vi "DequeueMessage.vi"(7 "Timeout (-1 ms)":i32=-1, 8 "error in":errorcluster, 11 "PriorityMessageQueue":refnum<class "PriorityMessageQueue.lvclass">) -> (0 "error out":errorcluster, 1 "Message out":refnum<class "Message.lvclass">, 2 "Message Name":string, 3 "PriorityMessageQueue out":refnum<class "PriorityMessageQueue.lvclass">, 4 "Timed Out?":bool)   [LabVIEW 2009, in "LapDog.Messaging.v2.lvlib" / "PriorityMessageQueue.lvclass"]
doc: "<b>This class is deprecated in version 2.1 and will be removed in version 3.0</b>\n\nDequeues a message object from the message queue. This vi does not output any errors on the error out terminal.\n\nIf the dequeue operation timeout expires a \"QueueTimeoutMessage\" Message object is sent.\nIf the dequeue operation generates an error the error cluster is bundled into a \"QueueErrorMessage\" ErrorMessage object and cleared from the wire. \nIf an error is on the input wire, the error cluster is bundled into a \"QueueErrorInMessage\" ErrorMessage object and cleared from the wire."
uses:
  PriorityMessageQueue.lvclass
  MessageObject/Message.lvclass
  ErrorMessage/ErrorMessage.lvclass
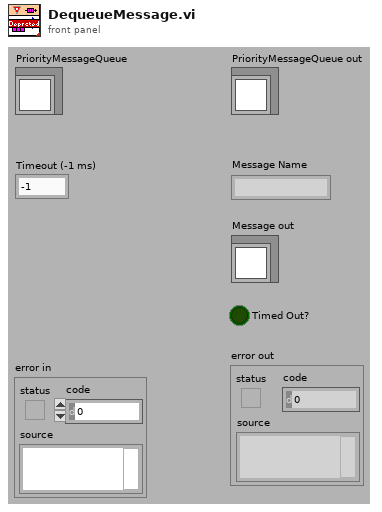
[diagram p1: front panel]
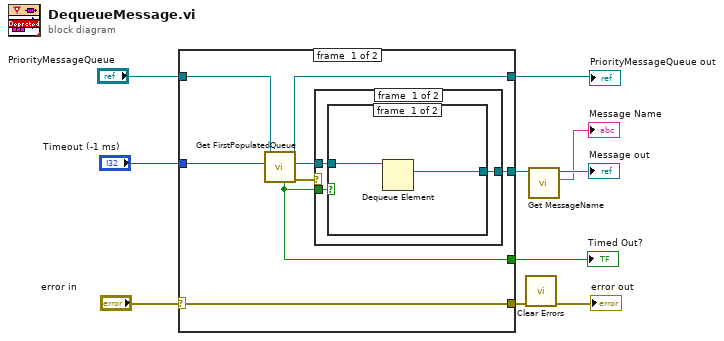
[diagram p0: block diagram]
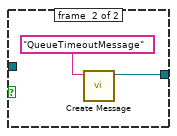
[diagram p2: hidden frame]
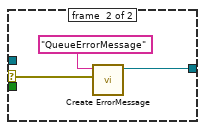
[diagram p3: hidden frame]
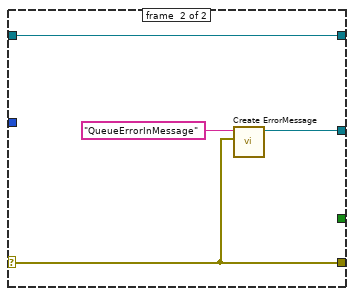
[diagram p4: hidden frame]
diagram:
  n1 = case shown="No Error" "error in" {
    selector: "error in" -> [w17 w30]
    tunnel: [w18 w31] -> w8
    tunnel: "Timeout (-1 ms)" -> [w14 _]
    tunnel: "PriorityMessageQueue" -> [w16 w32]
    tunnel: [w17 w30] -> w5
    tunnel: [w15 w32] -> w2
    tunnel: [w12 _] -> w1
    frame #0 {
      n2 = call "Get FirstPopulatedQueue.vi"("Timeout (-1 ms)"=w14, "PriorityMessageQueue in"=w16) -> ("error out"=w11:errorcluster, "MsgQ"=w13:refnum<queue>, "PriorityMessageQueue out"=w15:refnum<class "PriorityMessageQueue.lvclass">, "Timeout"=w12:bool)  [unwired: 6 in]
      n3 = case shown="Error" w11 {
        selector: w11 -> [_ w27]
        tunnel: [w20 w28] -> w18
        tunnel: w12 -> [w21 _]
        tunnel: w13 -> [w19 _]
        frame #0 {
          n4 = case shown="False" w21 {
            tunnel: [w22 w24] -> w20
            tunnel: w19 -> [w23 _]
            frame #0 {
              n5 = Dequeue Element(queue=w23) -> (element=w22:refnum<class "Message.lvclass">)  [unwired: 2 in, 3 out]
            }
            frame #1 {
              n6 = call "Create Message.vi"("Message Name"="QueueTimeoutMessage") -> ("Message out"=w24:refnum<class "Message.lvclass">)  [unwired: 9 in, 1 out]
            }
          }
        }
        frame #1 {
          n7 = call "Create ErrorMessage.vi"("Error Cluster"=w27, "Message Name"="QueueErrorMessage") -> ("ErrorMessage out"=w28:refnum<class "ErrorMessage.lvclass">)  [unwired: 8 in, 1 out]
        }
      }
    }
    frame #1 {
      n8 = call "Create ErrorMessage.vi"("Error Cluster"=w30, "Message Name"="QueueErrorInMessage") -> ("ErrorMessage out"=w31:refnum<class "ErrorMessage.lvclass">)  [unwired: 8 in, 1 out]
    }
  }
  "PriorityMessageQueue out" <- w2
  "Timed Out?" <- w1
  n9 = call <vilib>:"Clear Errors.vi"("error in (no error)"=w5) -> ("error out"=→"error out":errorcluster)  [unwired: 6 out]
  n10 = call "Get MessageName.vi"("Message in"=w8) -> ("Message Name"=→"Message Name":string, "Message out"=→"Message out":refnum<class "Message.lvclass">)  [unwired: 1 in, 8 out]
